vi "Hide Ctrl FGV.vi"(8 "error in (no error)":errorcluster, 9 "Hide":bool, 10 "Action":enum16{"Init", "Set Visibility"}(ring)=enum."Set Visibility", 11 "Controls Ref":refnum<vi>[](array[refnum])) -> (0 "error out":errorcluster)   [LabVIEW 2020, in "Protection and Counter Addon System Explorer.lvlib"]
uses:
  Protection and Counter Addon System Explorer.lvlib
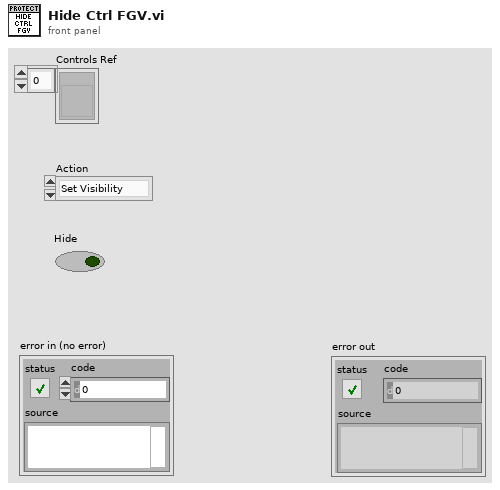
[diagram p1: front panel]
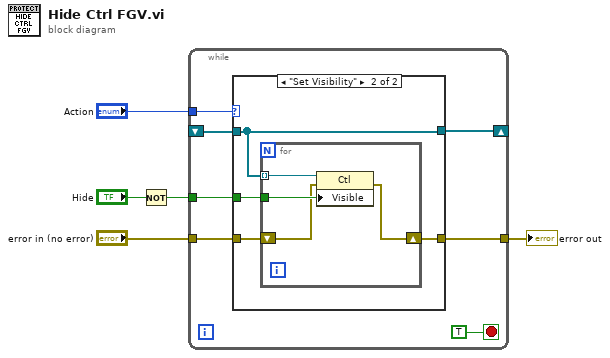
[diagram p0: block diagram]
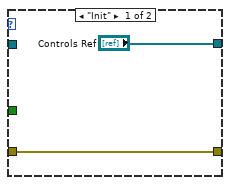
[diagram p2: hidden frame]
diagram:
  n1 = Not(x="Hide") -> (.not. x?=w3:bool)
  n2 = while {
    tunnel: "Action" -> [w12]
    shift-right: [w11] -> _
    shift-left: _ -> [w10]
    tunnel: w3 -> [w9]
    tunnel: "error in (no error)" -> [w8]
    tunnel: [w7] -> w1
    stop <- TRUE stop-if-true
    n3 = case shown="\"Set Visibility\"" w12 {
      tunnel: ["Controls Ref" w18] -> w11
      tunnel: w10 -> [_ w18]
      tunnel: w9 -> [_ w17]
      tunnel: w8 -> [w13 w16]
      tunnel: [w13 w15] -> w7
      frame "Init" {
      }
      frame "Set Visibility" {
        n4 = for {
          tunnel: w18 -> [w22] mode=indexing
          tunnel: w17 -> [w21]
          shift-right: [w19] -> w15
          shift-left: w16 -> [w20]
          n5 = property class="Ctl"(reference=w22, error in=w20, "Visible"=w21) -> (error out=w19:errorcluster)  [unwired: 1 out]
        }
      }
    }
  }
  "error out" <- w1
